vi "VI Tree.vi"   [LabVIEW 2022 SP3, in "Siglent SDG X Series.lvlib"]
doc: "This is the instrument driver for the Siglent SDG X series function(Pulse)/arbitrary generators. The VI Tree displays all the user-callable VIs of the instrument driver in an organized table."
uses:
  Siglent SDG X Series.lvlib
  Configure/Configure Modulation (AM).vi
panel:
  # "(c) 2017 SIGLENT TECHNOLOGIES CO.,LTD. ALL RIGHTS RESERVED."
  # "SEE DIAGRAM\nFOR VI TREE."
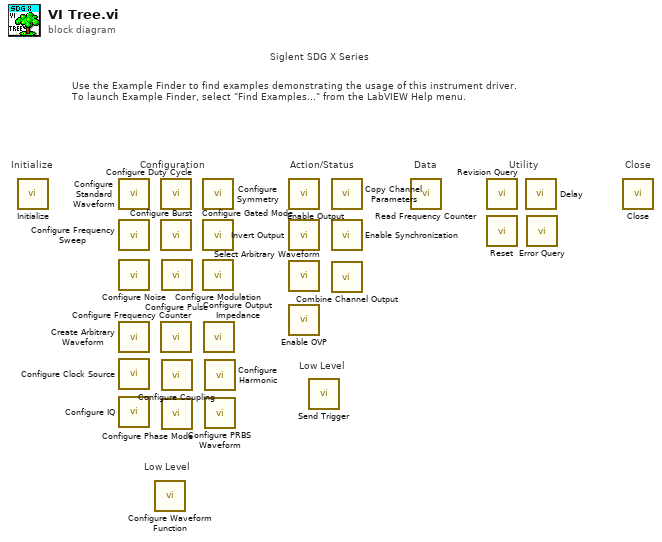
[diagram p0: block diagram]
diagram:
  # "Low Level"
  # "Siglent SDG X Series"
  # "Data"
  # "Low Level"
  # "Use the Example Finder to find examples demonstrating the usage of this instrument driver.\nTo launch Example Finder, select \"Find Examples...\" from the LabVIEW Help menu."
  # "Configuration"
  # "Utility"
  # "Action/Status"
  # "Close"
  # "Initialize"
  n1 = call "Initialize.vi"() -> ()  [unwired: 10 in, 2 out]
  n2 = call "Configure Standard Waveform.vi"() -> ()  [unwired: 14 in, 2 out]
  n3 = call "Configure Frequency Sweep.vi"() -> ()  [unwired: 14 in, 2 out]
  n4 = call "Configure Noise.vi"() -> ()  [unwired: 14 in, 2 out]
  n5 = call "Create Arbitrary Waveform.vi"() -> ()  [unwired: 10 in, 2 out]
  n6 = call "Configure Clock Source.vi"() -> ()  [unwired: 10 in, 2 out]
  n7 = call "Configure IQ.vi"() -> ()  [unwired: 14 in, 2 out]
  n8 = call "Configure Waveform Function.vi"() -> ()  [unwired: 10 in, 2 out]
  n9 = call "Configure Duty Cycle.vi"() -> ()  [unwired: 10 in, 2 out]
  n10 = call "Configure Burst.vi"() -> ()  [unwired: 18 in, 2 out]
  n11 = call "Configure Frequency Counter.vi"() -> ()  [unwired: 10 in, 2 out]
  n12 = call "Configure Pulse.vi"() -> ()  [unwired: 14 in, 2 out]
  n13 = call "Configure Coupling.vi"() -> ()  [unwired: 10 in, 2 out]
  n14 = call "Configure Phase Mode.vi"() -> ()  [unwired: 10 in, 2 out]
  n15 = call "Configure Symmetry.vi"() -> ()  [unwired: 10 in, 2 out]
  n16 = call "Configure Gated Mode.vi"() -> ()  [unwired: 14 in, 2 out]
  n17 = call-poly "Configure Modulation.vi"() -> ()  [unwired: 14 in, 2 out]
  n18 = call "Configure Output Impedance.vi"() -> ()  [unwired: 10 in, 2 out]
  n19 = call "Configure Harmonic.vi"() -> ()  [unwired: 14 in, 2 out]
  n20 = call "Configure PRBS Waveform.vi"() -> ()  [unwired: 14 in, 2 out]
  n21 = call "Enable Output.vi"() -> ()  [unwired: 10 in, 2 out]
  n22 = call "Invert Output.vi"() -> ()  [unwired: 10 in, 2 out]
  n23 = call "Select Arbitrary Waveform.vi"() -> ()  [unwired: 10 in, 2 out]
  n24 = call "Enable OVP.vi"() -> ()  [unwired: 10 in, 2 out]
  n25 = call "Send Trigger.vi"() -> ()  [unwired: 10 in, 2 out]
  n26 = call "Copy Channel Parameters.vi"() -> ()  [unwired: 10 in, 2 out]
  n27 = call "Enable Synchronization.vi"() -> ()  [unwired: 10 in, 2 out]
  n28 = call "Combine Channel Output.vi"() -> ()  [unwired: 10 in, 2 out]
  n29 = call "Read Frequency Counter.vi"() -> ()  [unwired: 9 in, 7 out]
  n30 = call "Revision Query.vi"() -> ()  [unwired: 8 in, 4 out]
  n31 = call "Reset.vi"() -> ()  [unwired: 10 in, 2 out]
  n32 = call "Delay.vi"() -> ()  [unwired: 10 in, 2 out]
  n33 = call "Error Query.vi"() -> ()  [unwired: 8 in, 4 out]
  n34 = call "Close.vi"() -> ()  [unwired: 11 in, 1 out]
